vi "MakePlotsNotWar.vi"(6 "transpose? (no:F)":bool, 10 "Channels to plot":T1, 11 "Data":dbl[][](array[numeric])) -> (1 "Y-axis names":string[](array[string]), 2 "X-axis name":string, 3 "Plots":cluster{"X Data":dbl[], "Y Data":dbl[]}[](array[cluster]), 4 "Y indexes":i32[](array[numeric]), 5 "X index":i32)   [LabVIEW 2015]
uses:
  Controls/Channels to plot.ctl
  Controls/Channel to plot.ctl
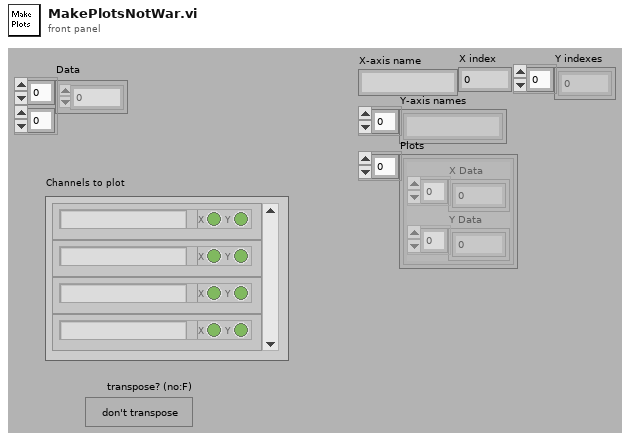
[diagram p1: front panel]
types:
  T1 = typedef "Channels to plot.ctl" = T2[]
  T2 = typedef "Channel to plot.ctl" = cluster{"Name":string, "X":bool, "Y":bool}
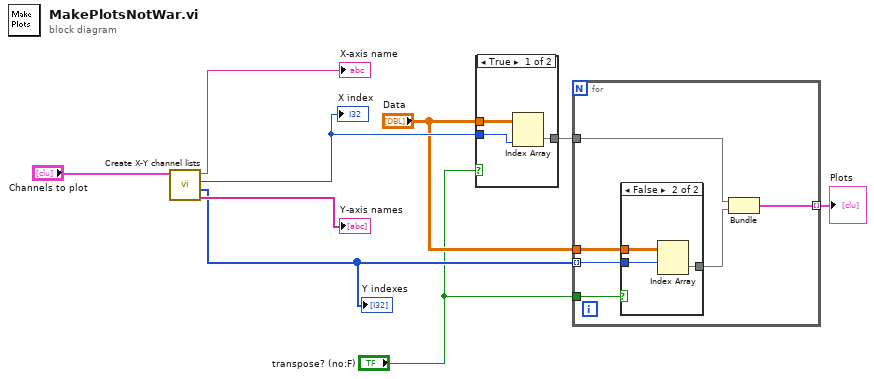
[diagram p0: block diagram]
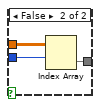
[diagram p2: hidden frame]
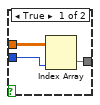
[diagram p3: hidden frame]
diagram:
  n1 = call "Create X-Y channel lists.vi"("Channels to plot"="Channels to plot") -> ("Y names"=→"Y-axis names":string[], "Y-axis indexes"=w7:i32[], "X index"=w6:i32, "X-axis name"=→"X-axis name":string)  [unwired: 6 in, 1 out]
  "X index" <- w6
  "Y indexes" <- w7
  n2 = case shown="True" "transpose? (no:F)" {
    tunnel: w6 -> [w10 w15]
    tunnel: "Data" -> [w12 w14]
    tunnel: [w11 w13] -> w4
    frame True {
      n3 = Index Array(array=w12, index (col)=w10) -> (element=w11:dbl[])  [unwired: 1 in]
    }
    frame False {
      n4 = Index Array(array=w14, index (row)=w15) -> (element=w13:dbl[])  [unwired: 1 in]
    }
  }
  n5 = for {
    tunnel: w7 -> [w19] mode=indexing
    tunnel: "Data" -> [w18]
    tunnel: w4 -> [w21]
    tunnel: [w20] -> w3 mode=indexing
    tunnel: "transpose? (no:F)" -> [w16]
    n6 = case shown="False" w16 {
      tunnel: w19 -> [w22 w27]
      tunnel: w18 -> [w24 w26]
      tunnel: [w23 w25] -> w17
      frame True {
        n7 = Index Array(array=w24, index (col)=w22) -> (element=w23:dbl[])  [unwired: 1 in]
      }
      frame False {
        n8 = Index Array(array=w26, index (row)=w27) -> (element=w25:dbl[])  [unwired: 1 in]
      }
    }
    n9 = Bundle("Data"=w21, "Data"=w17) -> (w20:cluster{"Data":dbl[], "Data":dbl[]})  [unwired: 1 out]
  }
  "Plots" <- w3
